vi "Mappa AO PLC_1.vi"(9 "Cluster":T1={"Scala profibus %lim. coppia max"=40.96, "Scala profibus %speed max"=163.84, "Scala profibus % coppia max"=40.96, "Scala profibus % V afe"=163.84, "Scala profibus % F afe"=163.84}, 10 "USCITE PLC":T2) -> (0 "Array DB REAL out":dbl[](array[numeric]), 1 "Array DB W out":dbl[](array[numeric]), 2 "Array M REAL out":dbl[](array[numeric]), 3 "Array M WORD out":dbl[](array[numeric]))   [LabVIEW 2019]
uses:
  Uscite PLC 1.ctl
  controls/statoAO_plc_1.ctl
  StatoDO_PLC_1.ctl
panel:
  # "StatoDO_PLC.ctlUSCITE PLC : TYPE DEF"
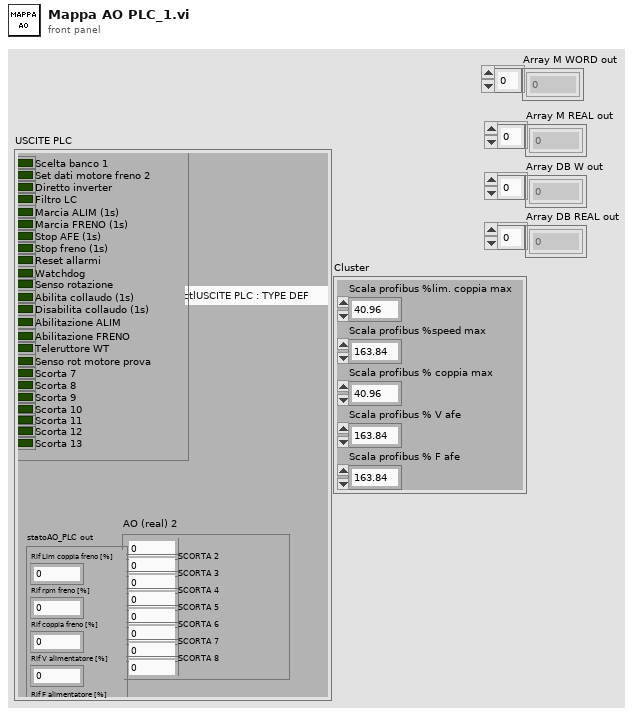
[diagram p1: front panel]
types:
  T1 = cluster{"Scala profibus %lim. coppia max":dbl, "Scala profibus %speed max":dbl, "Scala profibus % coppia max":dbl, "Scala profibus % V afe":dbl, "Scala profibus % F afe":dbl}
  T2 = typedef "Uscite PLC 1.ctl" = cluster{"AO (real) 2":cluster{"SCORTA 1":dbl, "SCORTA 2":dbl, "SCORTA 3":dbl, "SCORTA 4":dbl, "SCORTA 5":dbl, "SCORTA 6":dbl, "SCORTA 7":dbl, "SCORTA 8":dbl}, "statoAO_PLC out":T3, "DO (bit)":T4}
  T3 = typedef "statoAO_plc_1.ctl" = cluster{"Rif Lim coppia freno [%]":dbl, "Rif rpm freno [%]":dbl, "Rif coppia freno [%]":dbl, "Rif V alimentatore [%]":dbl, "Rif F alimentatore [%]":dbl}
  T4 = typedef "StatoDO_PLC_1.ctl" = cluster{"Scelta banco 1":bool, "Set dati motore freno 2":bool, "Diretto inverter":bool, "Filtro LC":bool, "Marcia ALIM (1s)":bool, "Marcia FRENO (1s)":bool, "Stop AFE (1s)":bool, "Stop freno (1s)":bool, "Reset allarmi":bool, "Watchdog":bool, "Senso rotazione":bool, "Abilita collaudo (1s)":bool, "Disabilita collaudo (1s)":bool, "Abilitazione ALIM":bool, "Abilitazione FRENO":bool, "Teleruttore WT":bool, "Senso rot motore prova":bool, "Scorta 7":bool, "Scorta 8":bool, "Scorta 9":bool, "Scorta 10":bool, "Scorta 11":bool, "Scorta 12":bool, "Scorta 13":bool}
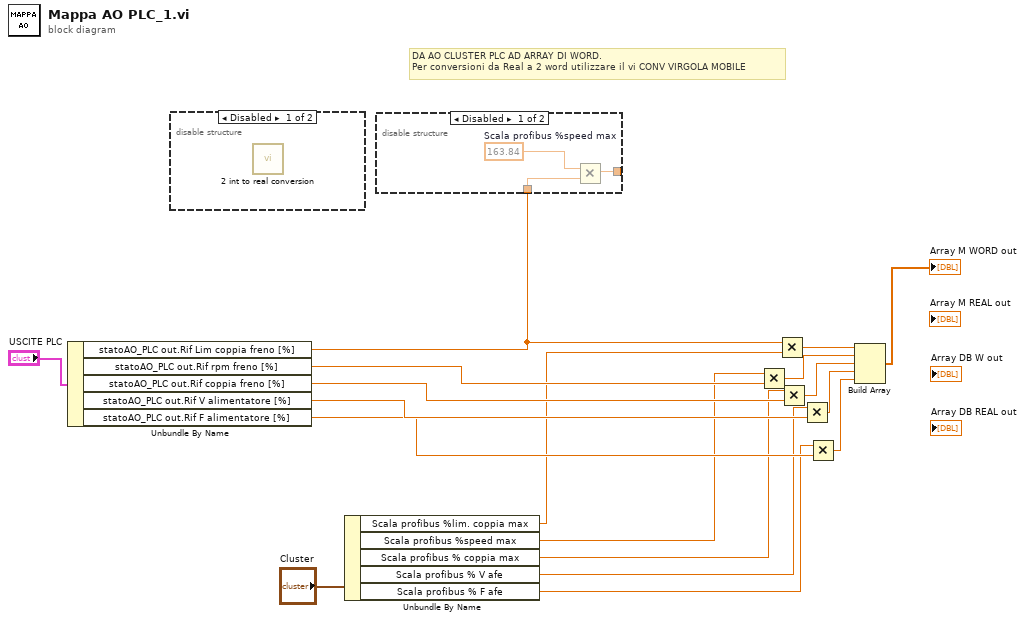
[diagram p0: block diagram]
diagram:
  # "DA AO CLUSTER PLC AD ARRAY DI WORD.\nPer conversioni da Real a 2 word utilizzare il vi CONV VIRGOLA MOBILE"
  n1 = Unbundle By Name("USCITE PLC") -> ("statoAO_PLC out.Rif Lim coppia freno [%]"=w16:dbl, "statoAO_PLC out.Rif rpm freno [%]"=w14:dbl, "statoAO_PLC out.Rif coppia freno [%]"=w12:dbl, "statoAO_PLC out.Rif V alimentatore [%]"=w11:dbl, "statoAO_PLC out.Rif F alimentatore [%]"=w10:dbl)
  n2 = disable-structure shown="Disabled" {
    frame Disabled {
      n3 = call "2 int to real conversion.vi"() -> ()  [unwired: 9 in, 3 out]
    }
    frame Enabled {
    }
  }
  n4 = Unbundle By Name("Cluster") -> ("Scala profibus %lim. coppia max"=w5:dbl, "Scala profibus %speed max"=w4:dbl, "Scala profibus % coppia max"=w3:dbl, "Scala profibus % V afe"=w2:dbl, "Scala profibus % F afe"=w1:dbl)
  n5 = disable-structure shown="Disabled" {
    disable-tunnel: w16 -> [w21 _]
    disable-tunnel: [w20 _] -> _
    frame Disabled {
      w19 = 163.84  # Scala profibus %speed max
      n6 = Multiply(x=w19, y=w21) -> (x*y=w20:dbl)
    }
    frame Enabled {
    }
  }
  n7 = Multiply(x=w4, y=w14) -> (x*y=w13:dbl)
  n8 = Multiply(x=w16, y=w5) -> (x*y=w15:dbl)
  n9 = Multiply(x=w3, y=w12) -> (x*y=w9:dbl)
  n10 = Multiply(x=w2, y=w11) -> (x*y=w8:dbl)
  n11 = Multiply(x=w1, y=w10) -> (x*y=w7:dbl)
  n12 = Build Array(w15, w13, w9, w8, w7) -> (→"Array M WORD out":dbl[])
